vi "GetPathReference.vi"(8 "error in":errorcluster, 11 "Path in":refnum<class "Path.lvclass">) -> (0 "error out":errorcluster, 1 "path reference":refnum<vi>, 3 "Path out":refnum<class "Path.lvclass">)   [LabVIEW 2014, in "Path.lvclass"]
uses:
  Path.lvclass
  Generic/Generic.lvclass
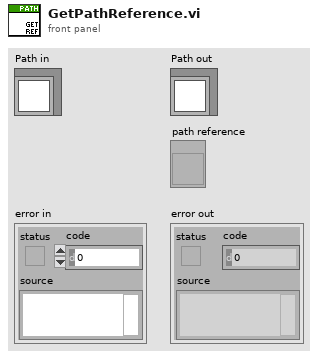
[diagram p1: front panel]
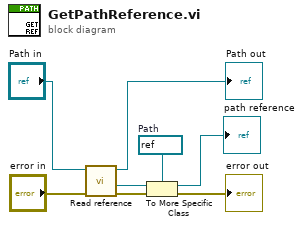
[diagram p0: block diagram]
diagram:
  w8 = refnum<vi> refnum  # Path
  n1 = call "Read reference.vi"("error in"="error in", "GObject in"="Path in") -> ("error out"=w5:errorcluster, "reference"=w4:refnum<vi>, "GObject out"=→"Path out":refnum<class "Path.lvclass">)  [unwired: 5 in]
  n2 = To More Specific Class(target class=w8, reference=w4, error in=w5) -> (specific class reference=→"path reference":refnum<vi>, error out=→"error out":errorcluster)
